vi "LR24ACircuit.vi"(7 "dt":dbl, 10 "voltage":dbl, 11 "curr_angle":dbl) -> (3 "angle":dbl)   [LabVIEW 2020]
doc: "Simulates the response of the LR24A actuator."
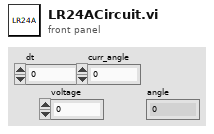
[diagram p1: front panel]
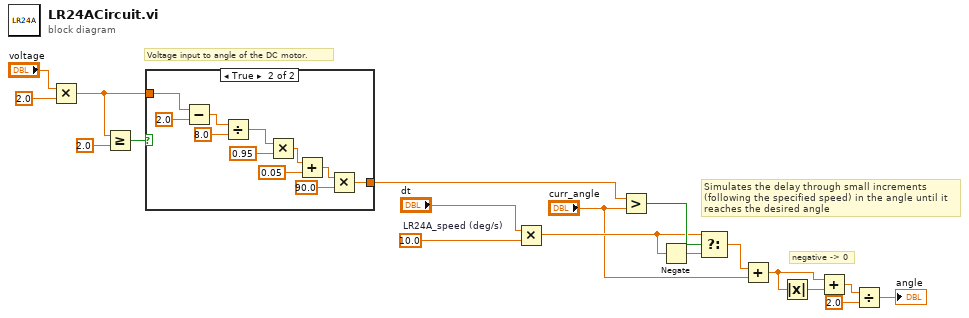
[diagram p0: block diagram]
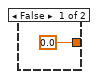
[diagram p2: hidden frame]
diagram:
  w11 = 10.0  # LR24A_speed (deg/s)
  # "Simulates the delay through small increments (following the specified speed) in the angle until it reaches the desired angle"
  # "Voltage input to angle of the DC motor."
  # "negative -> 0"
  n1 = Multiply(x="voltage", y=2.0) -> (x*y=w14:dbl)
  n2 = Greater Or Equal?(x=w14, y=2.0) -> (x >= y?=w16:bool)
  n3 = case shown="True" w16 {
    tunnel: [0.0 ("angle") w20] -> w7
    tunnel: w14 -> [_ w30]
    frame False {
    }
    frame True {
      n4 = Subtract(x=w30, y=2.0) -> (x-y=w28:dbl)
      n5 = Divide(x=w28, y=8.0) -> (x/y=w26:dbl)
      n6 = Multiply(x=w26, y=0.95) -> (x*y=w24:dbl)
      n7 = Add(x=w24, y=0.05) -> (x+y=w22:dbl)
      n8 = Multiply(x=w22, y=90.0) -> (x*y=w20:dbl)
    }
  }
  n9 = Multiply(x="dt", y=w11) -> (x*y=w8:dbl)
  n10 = Greater?(x=w7, y="curr_angle") -> (0:w13:bool)
  n11 = Negate(x=w8) -> (-x=w12:dbl)
  n12 = Select(t=w8, s=w13, f=w12) -> (s? t:f=w10:dbl)
  n13 = Add(x=w10, y="curr_angle") -> (x+y=w4:dbl)
  n14 = Absolute Value(x=w4) -> (abs(x)=w5:dbl)
  n15 = Add(x=w4, y=w5) -> (x+y=w3:dbl)
  n16 = Divide(x=w3, y=2.0) -> (x/y=→"angle":dbl)
